vi "Word Files.vi"(10 "error in":errorcluster, 11 "DesignRequest":T1) -> (2 "filenames":string[](array[string]), 3 "Word Files":path[](array[path]), 5 "error out":errorcluster)   [LabVIEW 2012]
uses:
  Design Request.ctl
  Variable cluster.ctl
  Folders.ctl
  Design Server.lvlib
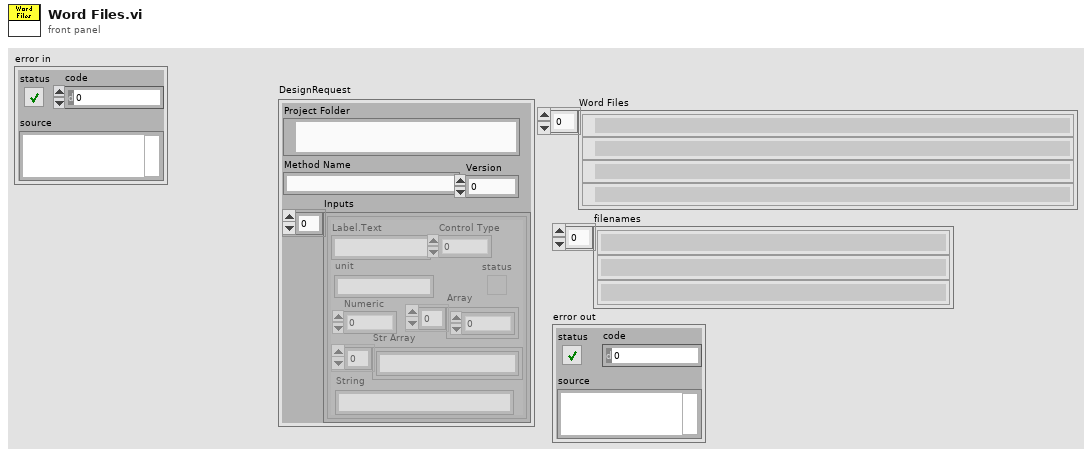
[diagram p1: front panel]
types:
  T1 = typedef "Design Server.lvlib/Design Request.ctl" = cluster{"Project Folder":path, "Method Name":string, "Inputs":T2, "Version":i32}
  T2 = typedef "Design Server.lvlib/Variable cluster.ctl" = cluster{"Label.Text":string, "Control Type":u32, "Numeric":dbl, "Array":dbl[], "status":bool, "Str Array":string[], "String":string, "unit":string}[]
  T3 = typedef "Design Server.lvlib/Folders.ctl" = enum16{"MathcadMethods", "RequestedDesigns", "CompletedDesigns", "MathcadCode", "CollabnetSVN.exe"}
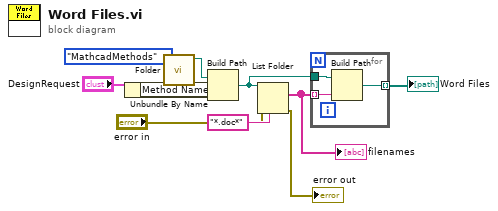
[diagram p0: block diagram]
diagram:
  n1 = Unbundle By Name("DesignRequest") -> ("Method Name"=w8:string)
  n2 = call "Folder.vi"("Folders"=Folders."MathcadMethods") -> ("FolderPath"=w7:path)  [unwired: 8 in, 2 out]
  n3 = Build Path(base path=w7, name or relative path=w8) -> (appended path=w4:path)
  n4 = List Folder(path=w4, pattern="*.doc*", error in="error in") -> (filenames=w5:string[], error out=→"error out":errorcluster)  [unwired: 1 in, 2 out]
  "filenames" <- w5
  n5 = for {
    tunnel: w5 -> [w13] mode=indexing
    tunnel: w4 -> [w12]
    tunnel: [w11] -> w3 mode=indexing
    n6 = Build Path(base path=w12, name or relative path=w13) -> (appended path=w11:path)
  }
  "Word Files" <- w3
